vi "rs3 get sensor count.vi"(8 "error in":errorcluster, 11 "sensor_list":u64) -> (0 "error out":errorcluster, 1 "sensor_list_out":u64, 2 "sensor count":i32, 3 "error":u64)   [LabVIEW 2017, in "libRealSense3.lvlib"]
doc: "Determines number of connected SENSORS\n \nerror non-null is an error\nreturn the count of devices"
uses:
  <vilib>/addons/RealSense/libRealSense3.lvlib
  Users/Greg McKaskle/Downloads/librealsense-1.12.1/librealsense-1.12.1/bin/Win32/realsense-d.dll
panel:
  # "RS3 Get Sensor Count"
  # "(C) Intel Corp.,  AGJ"
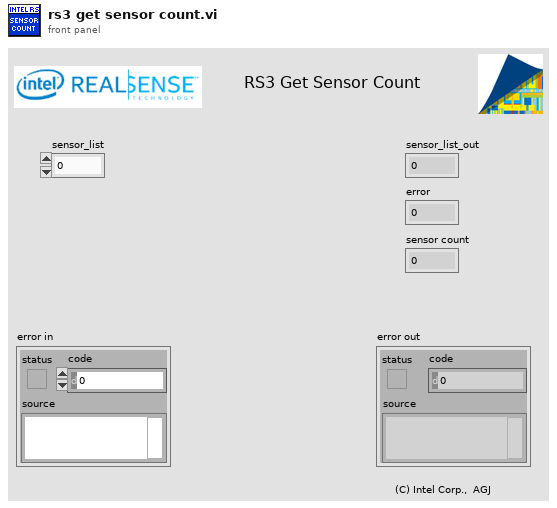
[diagram p1: front panel]
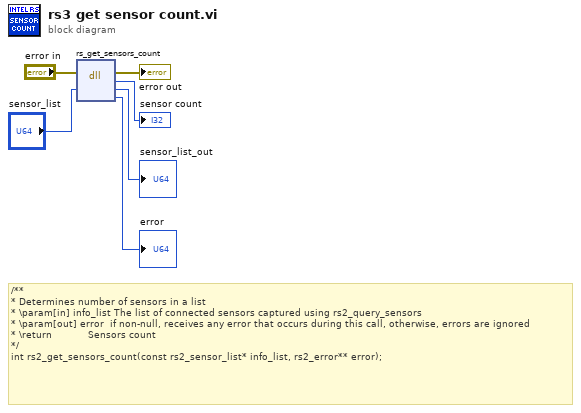
[diagram p0: block diagram]
diagram:
  # "/**\n* Determines number of sensors in a list\n* \\param[in] info_list The list of connected sensors captured using rs2_query_sensors\n* \\param[out] error  if non-null, receives any error that occurs during this call, otherwise, errors are ignored\n* \\return            Sensors count\n*/\nint rs2_get_sensors_count(const rs2_sensor_list* info_list, rs2_error** error);"
  n1 = dll-call lib="C:/Users/Greg McKaskle/Downloads/librealsense-1.12.1/librealsense-1.12.1/bin/Win32/realsense-d.dll" fn="rs_get_sensors_count"(error in="error in", "sensor list"="sensor_list") -> (error out=→"error out":errorcluster, "sensor count"=→"sensor count":i32, "sensor list"=→"sensor_list_out":u64, "error"=→"error":u64)  [unwired: 3 in, 1 out]
